vi "Collect Data1D.vi"(8 "error in (no error)":errorcluster, 10 "Data1D in":refnum<class "Data1D.lvclass">, 11 "AverageCollector1D in":refnum<class "AverageCollector1D.lvclass">) -> (0 "error out":errorcluster, 2 "finished?":bool=TRUE, 3 "AverageCollector1D out":refnum<class "AverageCollector1D.lvclass">)   [LabVIEW 2014, in "AverageCollector1D.lvclass"]
uses:
  AverageCollector1D.lvclass
  Framework/Model/Data/Data1D/Data1D.lvclass
  Framework/Collector/AbstractCollector/AbstractCollector.lvclass/AbstractCollector.ctl
  Framework/Collector/AbstractCollector/AbstractCollector.lvclass
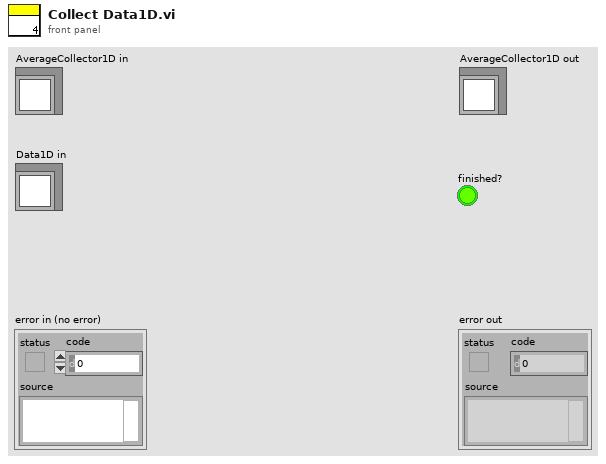
[diagram p1: front panel]
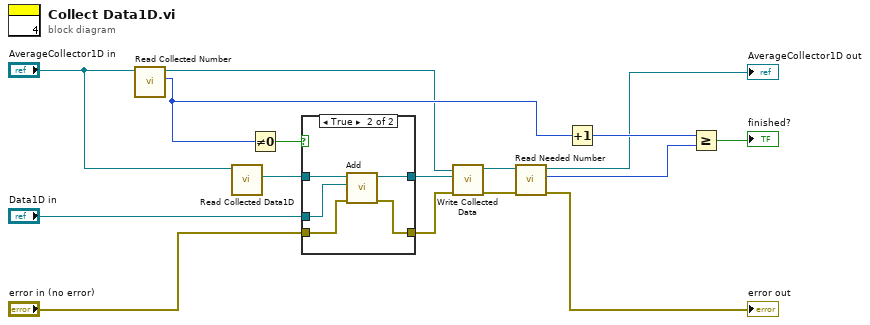
[diagram p0: block diagram]
diagram:
  n1 = call "Read Collected Number.vi"("AbstractCollector in"="AverageCollector1D in") -> ("collected"=w12:u32, "AbstractCollector out"=w4:refnum<class "AverageCollector1D.lvclass">)  [unwired: 8 in, 1 out]
  n2 = call-dynamic "Read Collected Data1D.vi"("AbstractCollector1D in"="AverageCollector1D in") -> ("Collected Data"=w1:refnum<class "Data1D.lvclass">)  [unwired: 8 in, 2 out]
  n3 = Not Equal To 0?(x=w12) -> (x != 0?=w11:bool)
  n4 = case shown="True" w11 {
    tunnel: [w17 w23] -> w10
    tunnel: [w18 w22] -> w9
    tunnel: "error in (no error)" -> [w18 w21]
    tunnel: w1 -> [_ w20]
    tunnel: "Data1D in" -> [w17 w19]
    frame False {
    }
    frame True {
      n5 = call-dynamic "Add.vi"("error in (no error)"=w21, "Data1D 2"=w19, "Data1D in"=w20) -> ("error out"=w22:errorcluster, "Data1D out"=w23:refnum<class "Data1D.lvclass">)  [unwired: 7 in]
    }
  }
  n6 = call-dynamic "Write Collected Data.vi"("error in (no error)"=w9, "Collected Data"=w10, "AbstractCollector in"=w4) -> ("error out"=w5:errorcluster, "AbstractCollector out"=w8:refnum<class "AverageCollector1D.lvclass">)  [unwired: 7 in]
  n7 = call-dynamic "Read Needed Number.vi"("error in (no error)"=w5, "AbstractCollector in"=w8) -> ("error out"=→"error out":errorcluster, "Needed Number"=w6:u32, "AbstractCollector out"=→"AverageCollector1D out":refnum<class "AverageCollector1D.lvclass">)  [unwired: 7 in]
  n8 = Increment(x=w12) -> (x+1=w13:u32)
  n9 = Greater Or Equal?(x=w13, y=w6) -> (x >= y?=→"finished?":bool)
